vi "Read Configuration.vi"(8 "error in":errorcluster) -> (0 "error out":errorcluster, 3 "Configuration":T1)   [LabVIEW 2020]
uses:
  <vilib>/Utility/config.llb/NI_LVConfig.lvlib
  Configuration--cluster.ctl
  <vilib>/Utility/config.llb/Read Key (String).vi
  <vilib>/Utility/config.llb/Read Key (Boolean).vi
  <vilib>/Utility/config.llb/Read Key (I32).vi
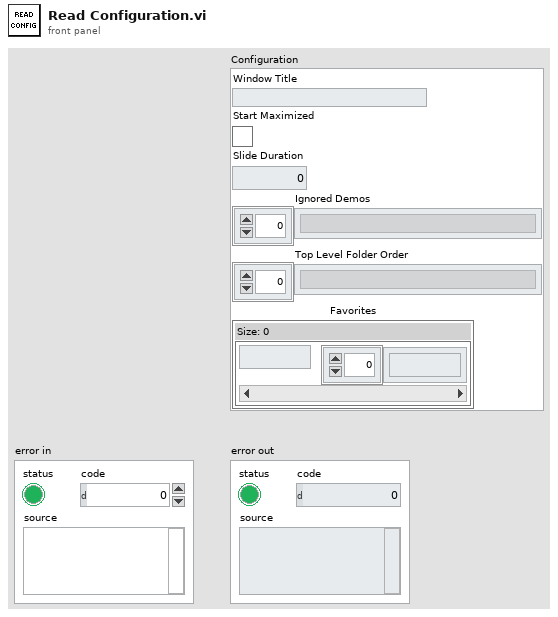
[diagram p1: front panel]
types:
  T1 = typedef "Configuration--cluster.ctl" = cluster{"Window Title":string, "Start Maximized":bool, "Slide Duration":i32, "Ignored Demos":string[], "Top Level Folder Order":string[], "Favorites":map{string, string[]}}
  T2 = typedef "NI_LVConfig.lvlib/Config Data RefNum.ctl" = refnum<k1>
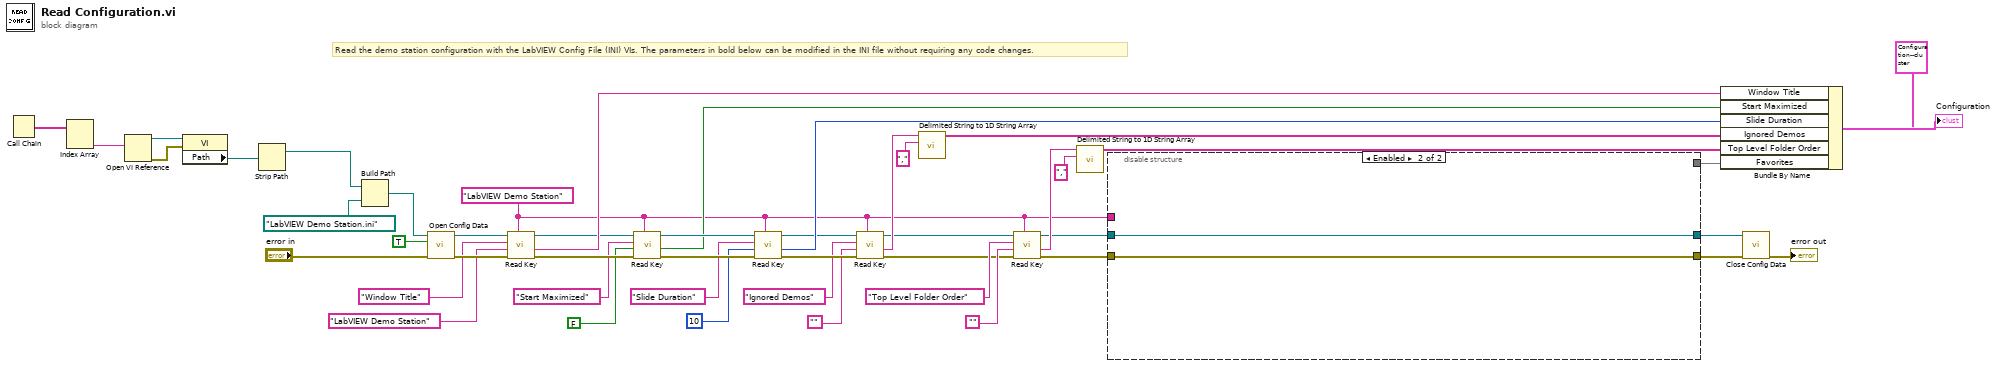
[diagram p0: block diagram]
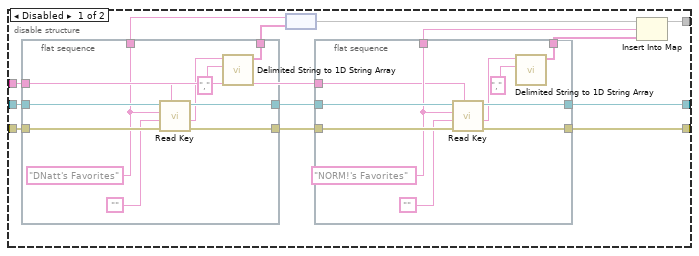
[diagram p2: hidden frame]
diagram:
  w8 = "LabVIEW Demo Station" ("section")
  # "Read the demo station configuration with the LabVIEW Config File (INI) VIs. The parameters in bold below can be modified in the INI file without requiring any code changes."
  n1 = Call Chain() -> (call chain=w6:string[])
  n2 = Index Array(array=w6) -> (element #2=w5:string)  [unwired: 2 in, 1 out]
  n3 = Open VI Reference(vi path=w5) -> (vi reference=w4:refnum<vi>, error out=w2:errorcluster)  [unwired: 5 in]
  n4 = property class="VI"(reference=w4, error in=w2) -> ("Path"=w3:path)  [unwired: 2 out]
  n5 = Strip Path(path=w3) -> (stripped path=w1:path)  [unwired: 1 out]
  n6 = Build Path(base path=w1, name or relative path=path "LabVIEW Demo Station.ini") -> (appended path=w46:path)
  n7 = call <vilib>:"Open Config Data.vi"("error in (no error)"="error in", "create file if necessary (T)"=TRUE, "configuration file path"=w46) -> ("error out"=w43:errorcluster, "refnum"=w42:T2)  [unwired: 6 in, 1 out]
  n8 = call-poly <vilib>:"Read Key.vi"("section"=w8, "error in (no error)"=w43, "default value"="LabVIEW Demo Station" ("section"), "key"="Window Title", "refnum"=w42) -> ("error out"=w37:errorcluster, "value"=w38:string, "refnum out"=w36:T2)  [unwired: 3 in, 1 out]
  n9 = call-poly <vilib>:"Read Key.vi"("section"=w8, "error in (no error)"=w37, "default value"=FALSE, "key"="Start Maximized", "refnum"=w36) -> ("error out"=w33:errorcluster, "value"=w30:bool, "refnum out"=w32:T2)  [unwired: 3 in, 1 out]
  n10 = call-poly <vilib>:"Read Key.vi"("section"=w8, "error in (no error)"=w33, "default value"=10, "key"="Slide Duration", "refnum"=w32) -> ("error out"=w26:errorcluster, "value"=w27:i32, "refnum out"=w25:T2)  [unwired: 3 in, 1 out]
  n11 = call-poly <vilib>:"Read Key.vi"("section"=w8, "error in (no error)"=w26, "default value"="", "key"="Ignored Demos", "refnum"=w25) -> ("error out"=w14:errorcluster, "value"=w23:string, "refnum out"=w15:T2)  [unwired: 3 in, 1 out]
  n12 = call <vilib>:"Delimited String to 1D String Array.vi"("delimiter"=",", "delimited string"=w23) -> ("string array"=w22:string[])  [unwired: 9 in]
  n13 = call-poly <vilib>:"Read Key.vi"("section"=w8, "error in (no error)"=w14, "default value"="", "key"="Top Level Folder Order", "refnum"=w15) -> ("error out"=w12:errorcluster, "value"=w17:string, "refnum out"=w11:T2)  [unwired: 3 in, 1 out]
  n14 = call <vilib>:"Delimited String to 1D String Array.vi"("delimiter"=",", "delimited string"=w17) -> ("string array"=w13:string[])  [unwired: 9 in]
  n15 = disable-structure shown="Enabled" {
    disable-tunnel: w12 -> [w61 w82]
    disable-tunnel: w11 -> [w60 w83]
    disable-tunnel: [w54 w83] -> w10
    disable-tunnel: [w53 w82] -> w9
    disable-tunnel: w8 -> [w52 _]
    disable-tunnel: [w51 _] -> w7
    frame Disabled {
      n16 = flat-sequence {
        tunnel: w61 -> [w81]
        tunnel: [w80] -> w55
        tunnel: w60 -> [w79]
        tunnel: [w78] -> w56
        tunnel: [w76] -> w59
        tunnel: [w73] -> w58
        tunnel: w52 -> [w72]
        frame #0 {
          w76 = "DNatt's Favorites" ("key")
          n17 = call-poly <vilib>:"Read Key.vi"("section"=w72, "error in (no error)"=w81, "default value"="", "key"=w76, "refnum"=w79) -> ("error out"=w80:errorcluster, "value"=w74:string, "refnum out"=w78:T2)  [unwired: 3 in, 1 out]
          n18 = call <vilib>:"Delimited String to 1D String Array.vi"("delimiter"=",", "delimited string"=w74) -> ("string array"=w73:string[])  [unwired: 9 in]
        }
      }
      n19 = node(w59, w58) -> (w57:map{string, string[]})
      n20 = flat-sequence {
        tunnel: w55 -> [w71]
        tunnel: [w70] -> w53
        tunnel: w56 -> [w69]
        tunnel: [w68] -> w54
        tunnel: [w66] -> w50
        tunnel: [w63] -> w49
        tunnel: w52 -> [w62]
        frame #0 {
          w66 = "NORM!'s Favorites" ("key")
          n21 = call-poly <vilib>:"Read Key.vi"("section"=w62, "error in (no error)"=w71, "default value"="", "key"=w66, "refnum"=w69) -> ("error out"=w70:errorcluster, "value"=w64:string, "refnum out"=w68:T2)  [unwired: 3 in, 1 out]
          n22 = call <vilib>:"Delimited String to 1D String Array.vi"("delimiter"=",", "delimited string"=w64) -> ("string array"=w63:string[])  [unwired: 9 in]
        }
      }
      n23 = Insert Into Map(map in=w57, key=w50, value=w49) -> (map out=w51:map{string, string[]})  [unwired: 2 out]
    }
    frame Enabled {
    }
  }
  n24 = Bundle By Name(cluster=T1 {"Window Title"="", "Start Maximized"=FALSE, "Slide Duration"=0, "Ignored Demos"=[], "Top Level Folder Order"=[], "Favorites"={}} ("Configuration"), "Window Title"=w38, "Start Maximized"=w30, "Slide Duration"=w27, "Ignored Demos"=w22, "Top Level Folder Order"=w13, "Favorites"=w7) -> (→"Configuration":T1)
  n25 = call <vilib>:"Close Config Data.vi"("error in (no error)"=w9, "refnum"=w10) -> ("error out"=→"error out":errorcluster)  [unwired: 8 in, 1 out]
